vi "WiggleMouse.vi"() -> ()   [LabVIEW 2014]
doc: "This VI is an event-driven loop that controls the wiggle timer timeout. This VI calls Mouse Wiggler driver to perform on-screen wiggle.\n\n**Author: Stas Legedza"
panel:
  in  "Stop":bool
  in  "Start":bool
  in  "Wiggle Timeout":T1={"Hours"=0, "Minutes"=0, "Seconds"=5} {"Seconds" min=5 max=60 step=1; "Minutes" max=60 step=1; "Hours" max=24 step=1}
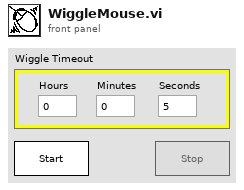
[diagram p1: front panel]
types:
  T1 = cluster{"Hours":u32, "Minutes":u32, "Seconds":u32}
  T2 = enum8{"Enabled", "Disabled", "Disabled and Grayed Out"}
  T3 = enum32{"invalid app kind", "Development System", "Run Time System", "Student Edition", "Embedded LabVIEW", "Evaluation", "Custom"}
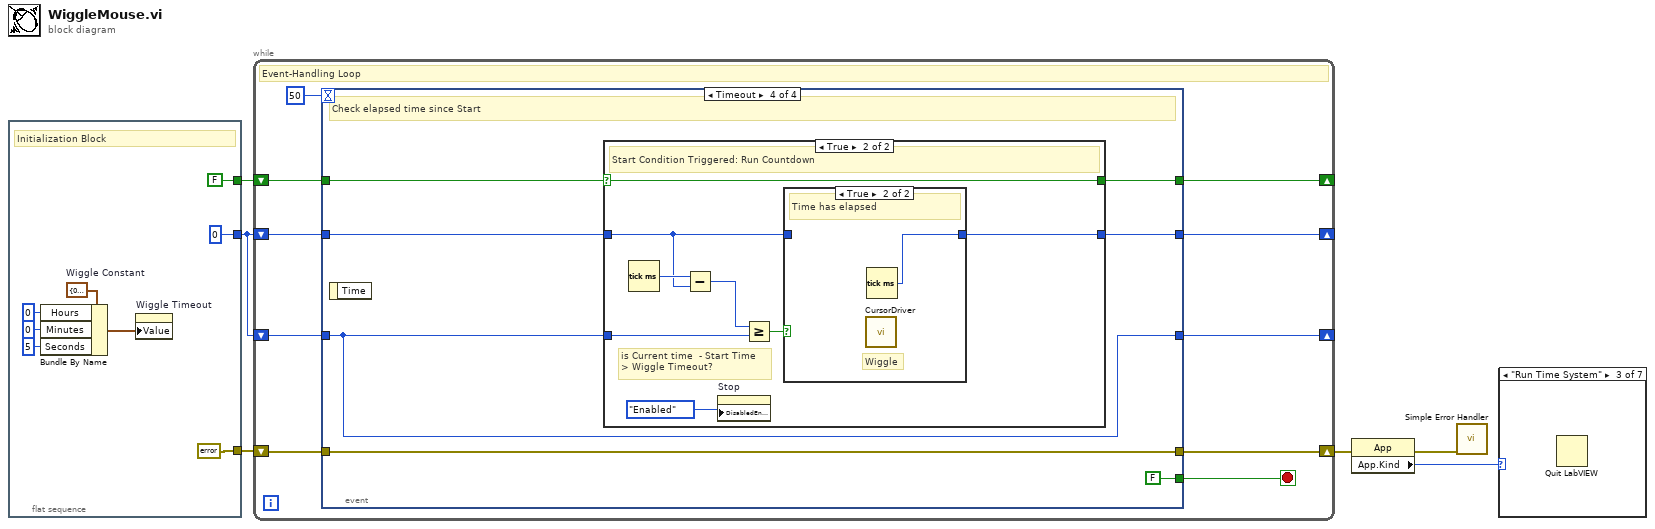
[diagram p0: block diagram]
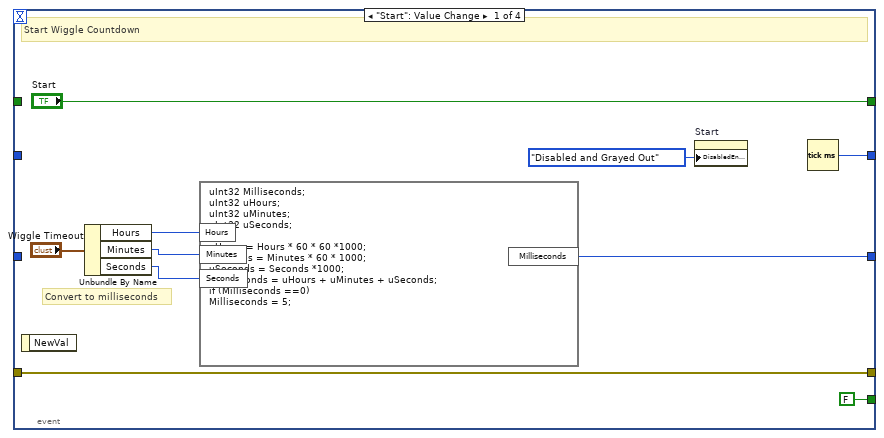
[diagram p8: hidden frame]
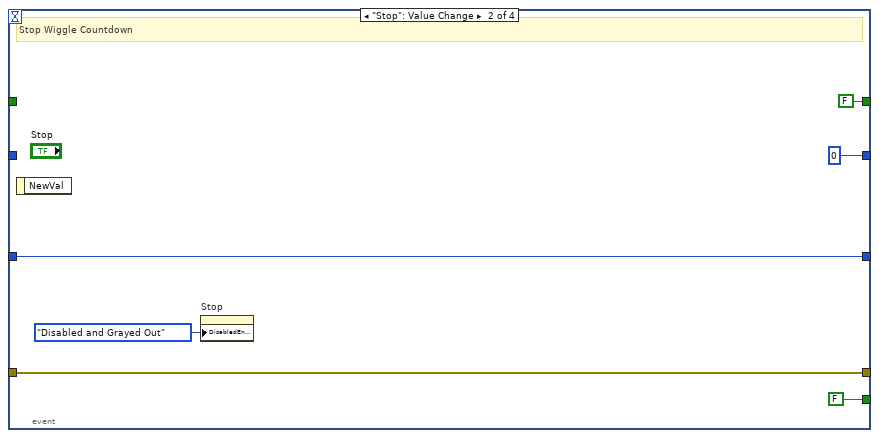
[diagram p9: hidden frame]
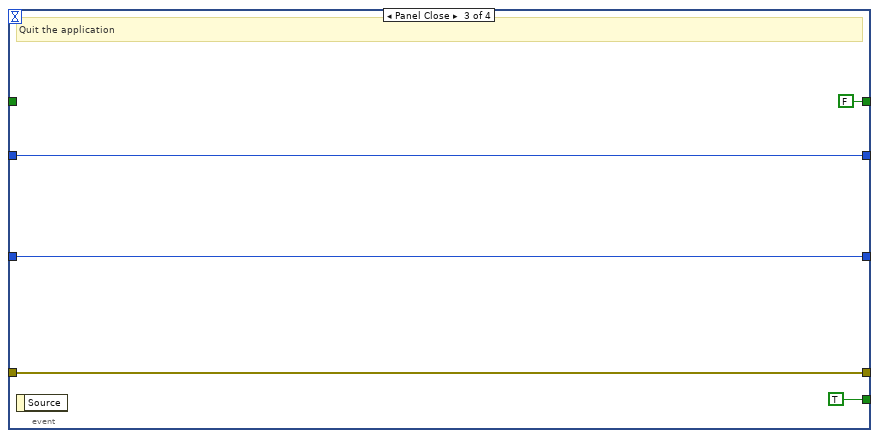
[diagram p10: hidden frame]
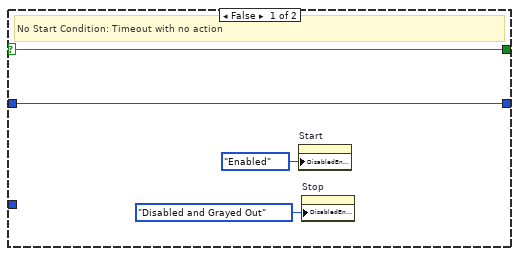
[diagram p11: hidden frame]
diagram:
  n1 = flat-sequence {
    tunnel: [u32 0 ("millisecond timer value")] -> w6
    tunnel: [errorcluster {"status"=FALSE, "code"=0, "source"=""} ("error in (no error)")] -> w5
    tunnel: [FALSE ("Start")] -> w1
    frame #0 {
      w12 = T1 {"Hours"=0, "Minutes"=0, "Seconds"=5}  # Wiggle Constant
      # "Initialization Block"
      n2 = Bundle By Name(cluster=w12, "Hours"=u32 0, "Minutes"=u32 0, "Seconds"=u32 5) -> (w8:T1)
      n3 = property on="Wiggle Timeout" class="Clust (strict)"("Value"=w8) -> ()  [unwired: 2 in, 2 out]
    }
  }
  n4 = while {
    shift-right: [w22] -> _
    shift-left: w6 -> [w21]
    shift-right: [w20] -> _
    shift-left: w6 -> [w19]
    shift-right: [w18] -> _
    shift-left: w1 -> [w17]
    shift-right: [w15] -> w4
    shift-left: w5 -> [w16]
    stop <- w23 stop-if-true
    # "Event-Handling Loop"
    n5 = event shown="[3] Timeout" {
      selector: _ -> [_ _ _ _]
      dyn-events: _ -> [_ _ _ _]
      timeout: 50 -> [_ _ _ _]
      tunnel: [FALSE FALSE TRUE FALSE] -> w23
      tunnel: [w32 u32 0 ("millisecond timer value") w45 w49] -> w22
      tunnel: w21 -> [_ _ w45 w50]
      tunnel: [w28 w36 w42 w51] -> w20
      tunnel: w19 -> [_ w36 w42 w51]
      tunnel: ["Start" FALSE ("Start") FALSE ("Start") w47] -> w18
      tunnel: w17 -> [_ _ _ w48]
      tunnel: w16 -> [w25 w35 w41 w46]
      tunnel: [w25 w35 w41 w46] -> w15
      event "Start": Value Change {
        # "Convert to milliseconds"
        # "Start Wiggle Countdown"
        n6 = event-data() -> ()  [unwired: 1 in, 1 out]
        n7 = Unbundle By Name("Wiggle Timeout") -> ("Hours"=w31:u32, "Minutes"=w30:u32, "Seconds"=w29:u32)
        n8 = formula code="uInt32 Milliseconds;\nuInt32 uHours;\nuInt32 uMinutes;\nuInt32 uSeconds;\n\nuHours = Hours * 60 * 60 *1000;\nuMinutes = Minutes * 60 * 1000;\nuSeconds = Seconds *1000;\nMilliseconds = uHours + uMinutes + uSeconds;\nif (Milliseconds ==0)\nMilliseconds = 5;"("Hours"=w31, "Minutes"=w30, "Seconds"=w29) -> ("Milliseconds"=w28:u32)
        n9 = property on="Start" class="Bool"("DisabledEnum"=T2."Disabled and Grayed Out" ("Disabled")) -> ()  [unwired: 2 in, 2 out]
        n10 = Tick Count (ms)() -> (millisecond timer value=w32:u32)
      }
      event "Stop": Value Change {
        # "Stop Wiggle Countdown"
        n11 = event-data() -> ()  [unwired: 1 in, 1 out]
        n12 = property on="Stop" class="Bool"("DisabledEnum"=T2."Disabled and Grayed Out" ("Disabled")) -> ()  [unwired: 2 in, 2 out]
      }
      event Panel Close {
        # "Quit the application"
        n13 = event-data() -> ()  [unwired: 1 in, 1 out]
      }
      event Timeout {
        # "Check elapsed time since Start"
        n14 = event-data() -> ()  [unwired: 1 in, 1 out]
        n15 = case shown="True" w48 {
          selector: w48 -> [w56 w58]
          tunnel: w51 -> [_ w61]
          tunnel: w50 -> [w55 w60]
          tunnel: [w55 w59] -> w49
          tunnel: [w56 w58] -> w47
          frame False {
            # "No Start Condition: Timeout with no action"
            n16 = property on="Start" class="Bool"("DisabledEnum"=T2."Enabled" ("Disabled")) -> ()  [unwired: 2 in, 2 out]
            n17 = property on="Stop" class="Bool"("DisabledEnum"=T2."Disabled and Grayed Out" ("Disabled")) -> ()  [unwired: 2 in, 2 out]
          }
          frame True {
            # "is Current time  - Start Time \n> Wiggle Timeout?"
            # "Start Condition Triggered: Run Countdown"
            n18 = Tick Count (ms)() -> (millisecond timer value=w64:u32)
            n19 = Subtract(x=w64, y=w60) -> (x-y=w63:u32)
            n20 = property on="Stop" class="Bool"("DisabledEnum"=T2."Enabled" ("Disabled")) -> ()  [unwired: 2 in, 2 out]
            n21 = Greater Or Equal?(x=w63, y=w61) -> (x >= y?=w62:bool)
            n22 = case shown="True" w62 {
              tunnel: w60 -> [w65 _]
              tunnel: [w65 w66] -> w59
              frame False {
                # "Time has not elapsed"
              }
              frame True {
                # "Wiggle"
                # "Time has elapsed"
                n23 = call "CursorDriver.vi"() -> ()  [unwired: 12 in]
                n24 = Tick Count (ms)() -> (millisecond timer value=w66:u32)
              }
            }
          }
        }
      }
    }
  }
  n25 = property class="App"(error in=w4) -> (error out=w3:errorcluster, "App.Kind"=w2:T3)  [unwired: 1 in, 1 out]
  n26 = call <vilib>:"Simple Error Handler.vi"("error in (no error)"=w3) -> ()  [unwired: 4 in, 5 out]
  n27 = case shown="\"Run Time System\"" w2 {
    frame "invalid app kind", Default {
    }
    frame "Development System" {
    }
    frame "Run Time System" {
      n28 = Quit LabVIEW() -> ()  [unwired: 1 in]
    }
    frame "Student Edition" {
    }
    frame "Embedded LabVIEW" {
    }
    frame "Evaluation" {
    }
    frame "Custom" {
    }
  }
